vi "CANOpen_Main_Start xPDOs.vi"(8 "error in (no error)":errorcluster, 10 "States":u16[](array[ring]) items=["unknown"=1, "bootup"=0, "stopped"=4, "operational"=5, "pre-operational"=127, "connection lost"=128], 11 "xPDO Refs":T1) -> (0 "error out":errorcluster)   [LabVIEW 2021, in "CANOpen Addon Engine.lvlib"]
uses:
  CANOpen Addon Engine.lvlib
  CANOpen_xPDO Refs.ctl
  CanOpen_RPDO Refs.ctl
  CanOpen_TPDO Refs.ctl
  <vilib>/CANopenLib/CANOPEN.llb/CANopen TPDO Start.vi
  <vilib>/CANopenLib/CANOPEN.llb/CANopen RPDO Start.vi
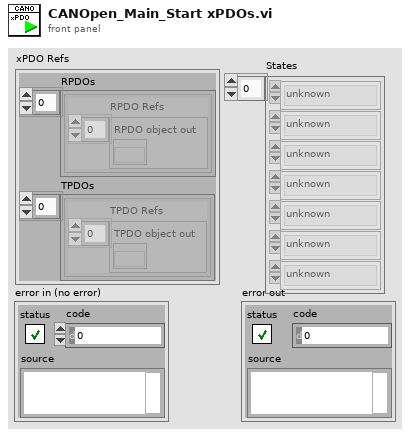
[diagram p1: front panel]
types:
  T1 = typedef "CANOpen Addon Engine.lvlib/CANOpen_xPDO Refs.ctl" = cluster{"RPDOs":T2[], "TPDOs":T3[]}
  T2 = typedef "CANOpen Addon Engine.lvlib/CanOpen_RPDO Refs.ctl" = cluster{"RPDO Refs":refnum<k20>[]}
  T3 = typedef "CANOpen Addon Engine.lvlib/CanOpen_TPDO Refs.ctl" = cluster{"TPDO Refs":refnum<k20>[]}
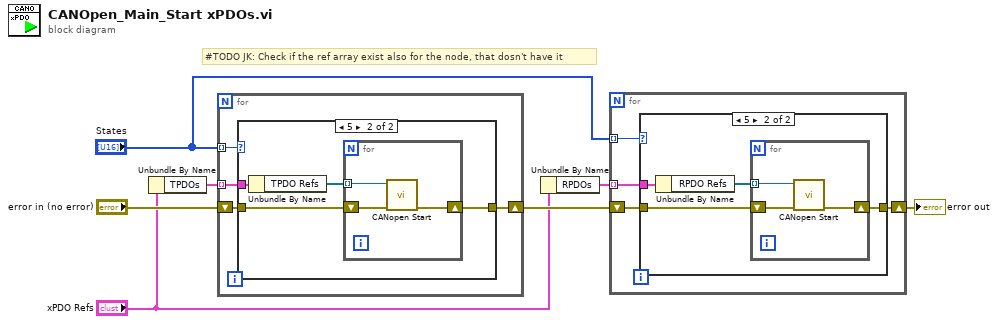
[diagram p0: block diagram]
diagram:
  # "#TODO JK: Check if the ref array exist also for the node, that dosn't have it"
  n1 = Unbundle By Name("xPDO Refs") -> ("TPDOs"=w6:T3[])
  n2 = for {
    tunnel: w6 -> [w9] mode=indexing
    shift-right: [w10] -> w5
    shift-left: "error in (no error)" -> [w11]
    tunnel: "States" -> [w8] mode=indexing
    n3 = case shown="5" w8 {
      tunnel: w11 -> [w12 w16]
      tunnel: [w12 w15] -> w10
      tunnel: w9 -> [_ w14]
      frame 0, Default {
      }
      frame 5 {
        n4 = Unbundle By Name(w14) -> ("TPDO Refs"=w13:refnum<k20>[])
        n5 = for {
          shift-right: [w18] -> w15
          shift-left: w16 -> [w19]
          tunnel: w13 -> [w17] mode=indexing
          n6 = call-poly <vilib>:"CANopen Start.vi"("error in (no error)"=w19, "TPDO object in"=w17) -> ("error out"=w18:errorcluster)  [unwired: 8 in, 1 out]
        }
      }
    }
  }
  n7 = Unbundle By Name("xPDO Refs") -> ("RPDOs"=w3:T2[])
  n8 = for {
    tunnel: w3 -> [w22] mode=indexing
    shift-right: [w20] -> w2
    shift-left: w5 -> [w23]
    tunnel: "States" -> [w21] mode=indexing
    n9 = case shown="5" w21 {
      tunnel: w23 -> [w24 w28]
      tunnel: w22 -> [_ w26]
      tunnel: [w24 w27] -> w20
      frame 0, Default {
      }
      frame 5 {
        n10 = Unbundle By Name(w26) -> ("RPDO Refs"=w25:refnum<k20>[])
        n11 = for {
          shift-right: [w30] -> w27
          shift-left: w28 -> [w31]
          tunnel: w25 -> [w29] mode=indexing
          n12 = call-poly <vilib>:"CANopen Start.vi"("error in (no error)"=w31, "RPDO object in"=w29) -> ("error out"=w30:errorcluster)  [unwired: 8 in, 1 out]
        }
      }
    }
  }
  "error out" <- w2
